vi "Controller & output.vi"() -> ()   [LabVIEW 2016]
doc: "Manually blink and LED attached to a digital output channel of a LINX device by clicking and LED control in LabVIEW."
uses:
  <vilib>/MakerHub/Xbox-One-Controller/Private/Type Defs/Indicators/Controller.ctl
  <vilib>/MakerHub/Xbox-One-Controller/Private/Type Defs/Indicators/A.ctl
  <vilib>/MakerHub/Xbox-One-Controller/Private/Type Defs/Indicators/B.ctl
  <vilib>/MakerHub/Xbox-One-Controller/Private/Type Defs/Indicators/X.ctl
  <vilib>/MakerHub/Xbox-One-Controller/Private/Type Defs/Indicators/Y.ctl
  <vilib>/MakerHub/Xbox-One-Controller/Private/Type Defs/Indicators/Left Bumper.ctl
  <vilib>/MakerHub/Xbox-One-Controller/Private/Type Defs/Indicators/Right Bumper.ctl
  <vilib>/MakerHub/Xbox-One-Controller/Private/Type Defs/Indicators/View.ctl
  <vilib>/MakerHub/Xbox-One-Controller/Private/Type Defs/Indicators/Menu.ctl
  <vilib>/MakerHub/Xbox-One-Controller/Private/Type Defs/Indicators/Thumbstick_Analog.ctl
  <vilib>/MakerHub/Xbox-One-Controller/Private/Type Defs/Indicators/Slider.ctl
  <vilib>/MakerHub/Xbox-One-Controller/Private/Type Defs/Indicators/DPad.ctl
  <vilib>/MakerHub/LINX/Public/Peripherals/Digital/Digital Write 1 Chan.vi
  <vilib>/MakerHub/LINX/Public/Peripherals/Digital/Digital Write N Chans.vi
  <vilib>/MakerHub/LINX/Private/Local IO/LinxDigitalWrite.vi
  <vilib>/MakerHub/LINX/Public/Utilities/Check Channel.vi
  <vilib>/MakerHub/LINX/Public/Utilities/Open Serial.vi
  <vilib>/MakerHub/Xbox-One-Controller/Public/Open First Controller.vi
  <vilib>/MakerHub/LINX/Private/Utilties/Generate Error.vi
  <vilib>/MakerHub/LINX/LMH-LINX.lvlib
  <vilib>/MakerHub/Xbox-One-Controller/LMH-Xbox-One-Controller.lvlib
panel:
  in  "Brake":bool
  in  "DO Channel 2":u8
  in  "y":i32
  out "element":i32
  out "Y Value":i32[](array[numeric])
  out "X value":i32[](array[numeric])
  out "Left Stick":T1
  in  "Frequency (Hz)":u32
  in  "Duration (ms)":u32
  in  "PWM Channel":u8=13
  in  "Stop Button 2":bool
  out "Controller":T2={"A Button"=FALSE, "B Button"=FALSE, "X Button"=FALSE, "Y Button"=FALSE, "Left Bumper"=FALSE, "Right Bumper"=FALSE, "View Button"=FALSE, "Menu Button"=FALSE, "Left Stick"={[], []}, "Right Stick"={[], []}, "Trigger"=0, "D-Pad"=5} {"Trigger" scale=32767.0..-32768.0}
  out "Loop Rate (Hz)":u32
  in  "LED Value":bool
  in  "Digital Output Channel":u8=13
  in  "Serial Port":refnum<visa-resource-name>
  in  "Stop Button":bool
  # "Circuit Schematic"
  # "LINX Device Settings"
  # "Direction"
  # "Manual Blink Example\n\nThis example demonstrates how to blink an LED on a LINX device by clicking on an LED control in LabVIEW.\n\nInstructions\n1. Select the Serial Port associated with the LINX Device.\n2. Select the Digital Output Channel connected to the LED.\n3. Click the Run Arrow."
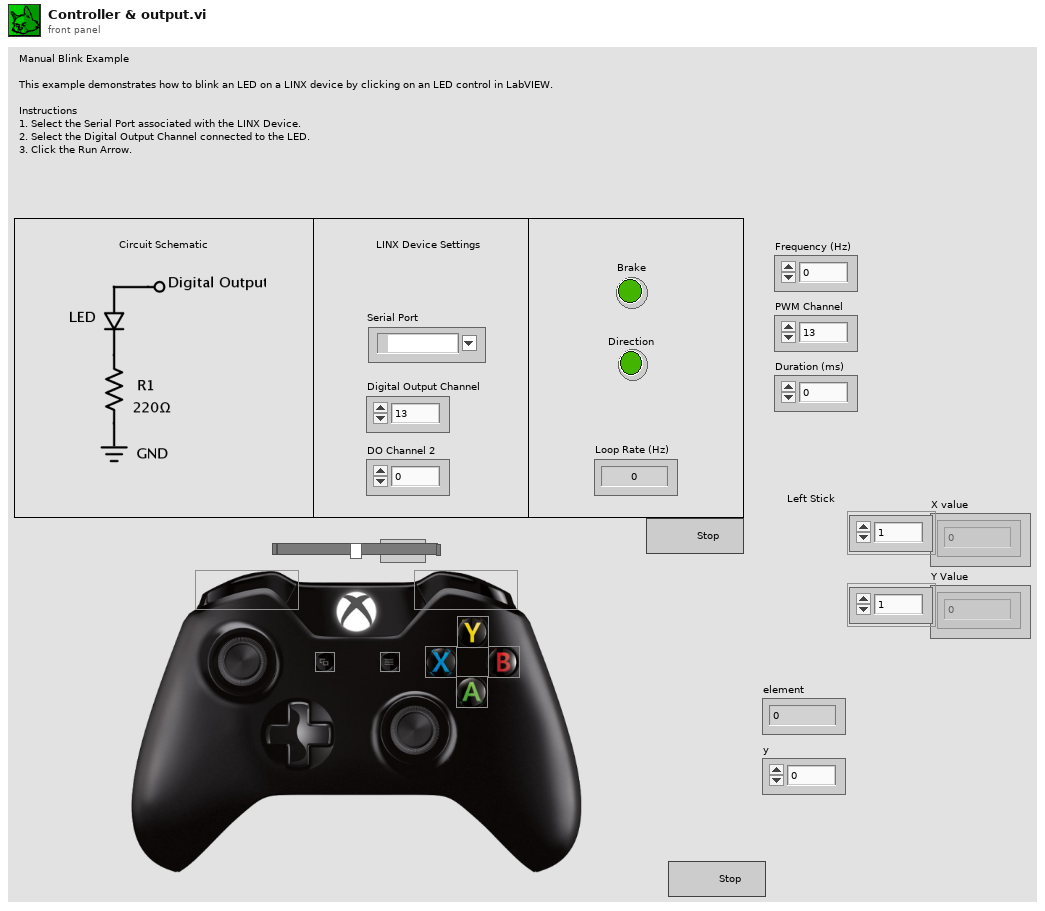
[diagram p1: front panel]
types:
  T1 = typedef "LMH-Xbox-One-Controller.lvlib/Thumbstick_Analog.ctl" = cluster{i32[], i32[]}
  T2 = typedef "LMH-Xbox-One-Controller.lvlib/Controller.ctl" = cluster{"A Button":T3, "B Button":T4, "X Button":T5, "Y Button":T6, "Left Bumper":T7, "Right Bumper":T8, "View Button":T9, "Menu Button":T10, "Left Stick":T1, "Right Stick":T1, "Trigger":T11, "D-Pad":T12}
  T3 = typedef "LMH-Xbox-One-Controller.lvlib/A.ctl" = bool
  T4 = typedef "LMH-Xbox-One-Controller.lvlib/B.ctl" = bool
  T5 = typedef "LMH-Xbox-One-Controller.lvlib/X.ctl" = bool
  T6 = typedef "LMH-Xbox-One-Controller.lvlib/Y.ctl" = bool
  T7 = typedef "LMH-Xbox-One-Controller.lvlib/Left Bumper.ctl" = bool
  T8 = typedef "LMH-Xbox-One-Controller.lvlib/Right Bumper.ctl" = bool
  T9 = typedef "LMH-Xbox-One-Controller.lvlib/View.ctl" = bool
  T10 = typedef "LMH-Xbox-One-Controller.lvlib/Menu.ctl" = bool
  T11 = typedef "LMH-Xbox-One-Controller.lvlib/Slider.ctl" = i32
  T12 = typedef "LMH-Xbox-One-Controller.lvlib/DPad.ctl" = u16
  T13 = typedef "LMH-LINX.lvlib/LINX Ref.ctl" = cluster{"IO":T14, "Interface":T15, "LINX Device Config":T16}
  T14 = typedef "LMH-LINX.lvlib/Platform.ctl" = enum16{"Remote", "Local"}
  T15 = typedef "LMH-LINX.lvlib/Interface.ctl" = enum16{"Serial", "TCP"}
  T16 = typedef "LMH-LINX.lvlib/Device.lvlib/LINX Device Config.ctl" = cluster{"Interface":T15, "COM Port":refnum<visa-resource-name>, "TCP Configuration":T17, "Device Family":u8, "Device ID":u8, "Device Name":string, "TCP Ref":refnum<k5>, "Channels":T18}
  T17 = typedef "LMH-LINX.lvlib/Device.lvlib/TCP Config.ctl" = cluster{"IP Address":string, "Port":u16}
  T18 = typedef "LMH-LINX.lvlib/Channels.ctl" = cluster{"DI":u8[], "DO":u8[], "AI":u8[], "AO":u8[], "PWM":u8[], "QE":u8[], "UART":u8[], "I2C 2":u8[], "SPI":u8[], "CAN":u8[], "Servo":u8[], "AI Ref (V)":dbl, "AI Resolution (Bits)":u8, "AO Ref (V)":dbl, "AO Resolution (Bits)":u8}
  T19 = typedef "LMH-Xbox-One-Controller.lvlib/Xbox One Controller Ref.ctl" = cluster{"Controller Ref":refnum<k1>, "Event Refnum":refnum<event-registration>, "Worker Ref":refnum<vi>}
  T20 = typedef "LMH-Xbox-One-Controller.lvlib/All Axis Data.ctl" = cluster{"Left Stick":cluster{"X Axis":i32, "Y Axis":i32}, "Right Stick":cluster{"X Axis":i32, "Y Axis":i32}, "Triggers":i32, "D-Pad":T21}
  T21 = typedef "LMH-Xbox-One-Controller.lvlib/DPad Enum.ctl" = enum16{"Idle", "Up", "Up / Right", "Right", "Down / Right", "Down", "Down / Left", "Left", "Up / Left"}
  T22 = typedef "LMH-Xbox-One-Controller.lvlib/All Buttons Visual.ctl" = cluster{"A":T3, "B":T4, "X":T5, "Y":T6, "Left Bumper":T7, "Right Bumper":T8, "View Button":T9, "Menu Button":T10, "Left Stick":T23, "Right Stick":T23}
  T23 = typedef "LMH-Xbox-One-Controller.lvlib/Thumbstick.ctl" = bool
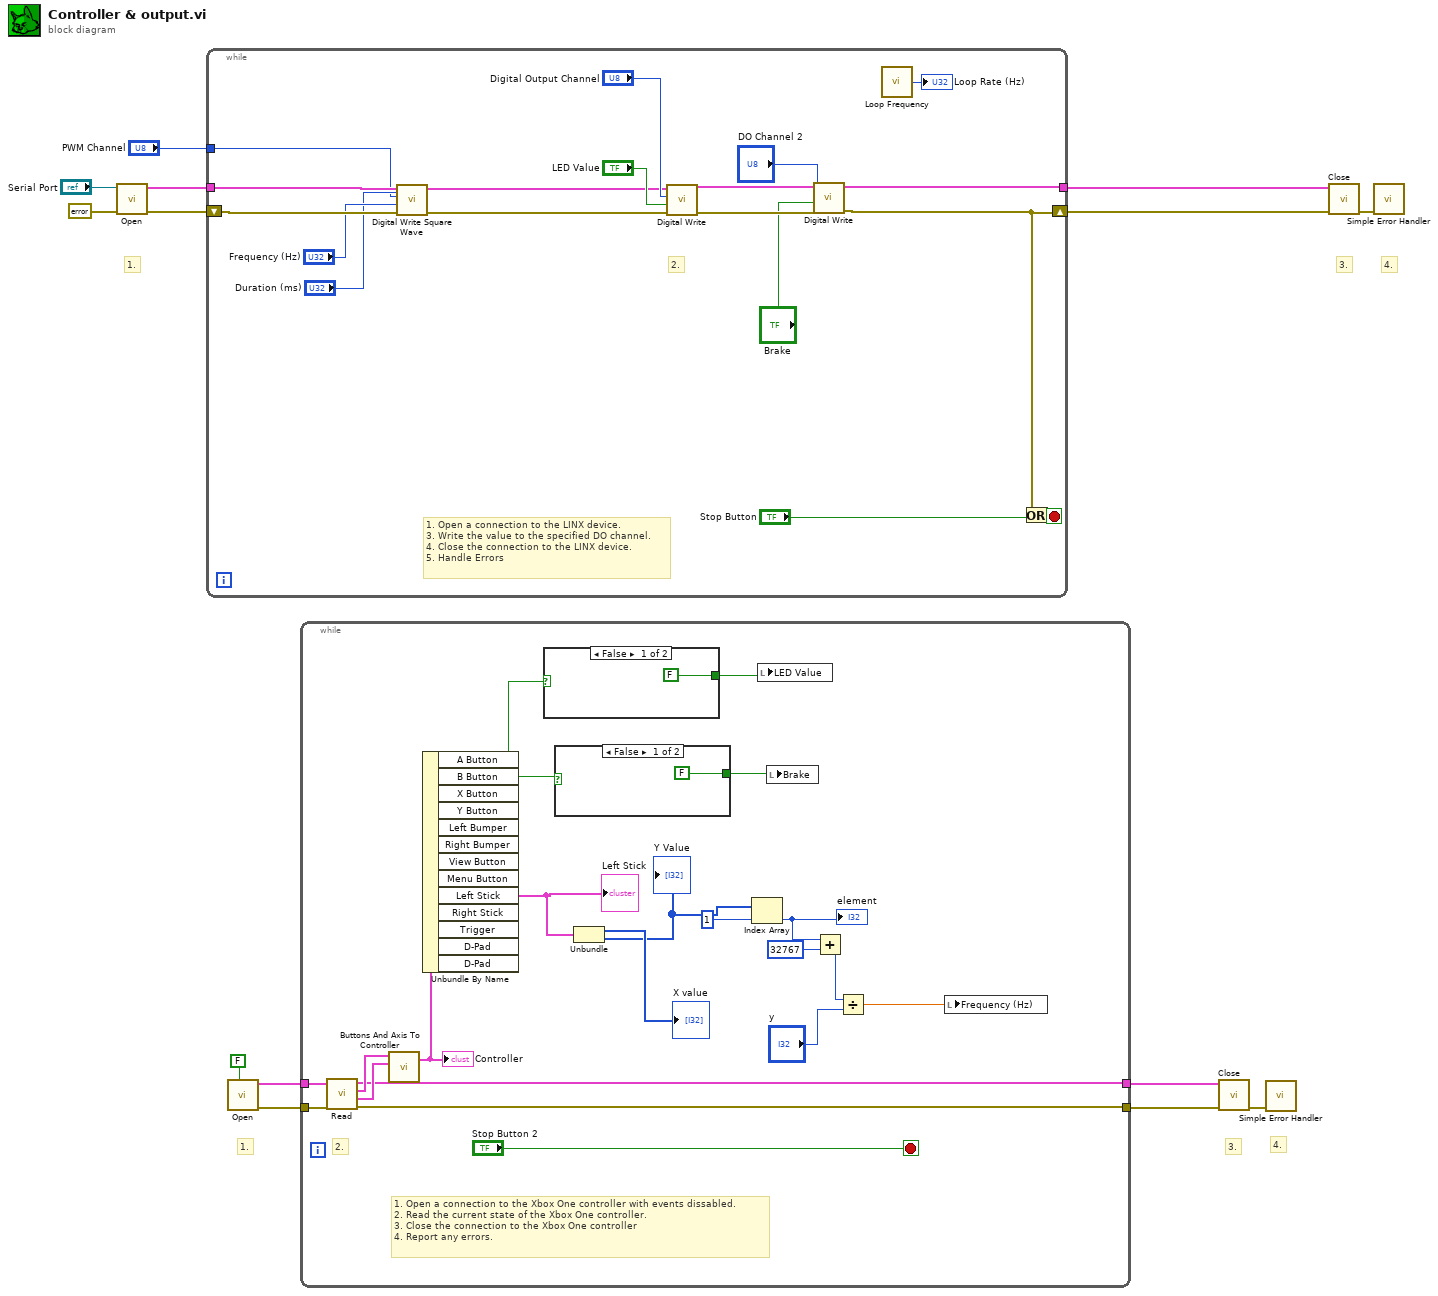
[diagram p0: block diagram]
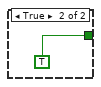
[diagram p2: hidden frame]
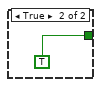
[diagram p3: hidden frame]
diagram:
  # "4."
  # "3."
  # "1."
  # "4."
  # "3."
  # "1."
  n1 = call-poly <vilib>:"Open.vi"("Error In"=errorcluster {"status"=FALSE, "code"=0, "source"=""}, "Serial Port"="Serial Port") -> ("Error Out"=w13:errorcluster, "LINX Resource"=w14:T13)  [unwired: 7 in, 1 out]
  n2 = while {
    tunnel: w14 -> [w24]
    tunnel: [w20] -> w12
    shift-right: [w17] -> w11
    shift-left: w13 -> [w25]
    tunnel: "PWM Channel" -> [w21]
    stop <- w32 stop-if-true
    # "1. Open a connection to the LINX device.\n3. Write the value to the specified DO channel.\n4. Close the connection to the LINX device.\n5. Handle Errors"
    # "2."
    n3 = call <vilib>:"Digital Write Square Wave.vi"("Duration (ms)"="Duration (ms)", "Error In"=w25, "Frequency (Hz)"="Frequency (Hz)", "Channel"=w21, "LINX Resource"=w24) -> ("Error Out"=w26:errorcluster, "LINX Resource"=w27:T13)  [unwired: 5 in]
    n4 = call-poly <vilib>:"Digital Write.vi"("Error In"=w26, "Output Value"="LED Value", "DO Channel"="Digital Output Channel", "LINX Resource"=w27) -> ("Error Out"=w18:errorcluster, "LINX Resource"=w19:T13)  [unwired: 6 in]
    n5 = call-poly <vilib>:"Digital Write.vi"("Error In"=w18, "Output Value"="Brake", "DO Channel"="DO Channel 2", "LINX Resource"=w19) -> ("Error Out"=w17:errorcluster, "LINX Resource"=w20:T13)  [unwired: 6 in]
    n6 = call <vilib>:"Loop Frequency.vi"() -> ("Loop Rate (Hz)"=→"Loop Rate (Hz)":u32)
    n7 = Or(x=w17, y="Stop Button") -> (x .or. y?=w32:bool)
  }
  n8 = call-poly <vilib>:"Open.vi"("Enable Events (T)"=FALSE) -> ("Error Out"=w5:errorcluster, "Xbox One Controller"=w6:T19)  [unwired: 8 in, 1 out]
  n9 = while {
    tunnel: w5 -> [w52]
    tunnel: w6 -> [w47]
    tunnel: [w49] -> w2
    tunnel: [w48] -> w3
    stop <- "Stop Button 2" stop-if-true
    # "1. Open a connection to the Xbox One controller with events dissabled.\n2. Read the current state of the Xbox One controller.\n3. Close the connection to the Xbox One controller\n4. Report any errors."
    # "2."
    n10 = call <vilib>:"Read.vi"("Error In"=w52, "Xbox One Controller Ref"=w47) -> ("Error Out"=w48:errorcluster, "All Axis"=w50:T20, "Buttons"=w51:T22, "Xbox One Controller Ref"=w49:T19)  [unwired: 6 in]
    n11 = call <vilib>:"Buttons And Axis To Controller.vi"("All Axis"=w50, "Buttons"=w51) -> ("Controller"=w46:T2)  [unwired: 5 in]
    "Controller" <- w46
    n12 = Unbundle By Name(w46) -> ("A Button"=w45:T3, "B Button"=w33:T4, "Left Stick"=w43:T1)  [unwired: 10 out]
    "Left Stick" <- w43
    n13 = case shown="False" w45 {
      tunnel: [FALSE ("LED Value") TRUE ("LED Value")] -> w44
      frame False {
      }
      frame True {
      }
    }
    n14 = case shown="False" w33 {
      tunnel: [FALSE ("LED Value") TRUE ("LED Value")] -> w34
      frame False {
      }
      frame True {
      }
    }
    n15 = Unbundle(w43) -> (→"X value":i32[], w41:i32[])
    "Y Value" <- w41
    n16 = Index Array(array=w41, index=1) -> (element=w37:i32)
    "element" <- w37
    n17 = local write "LED Value"(w44) -> ()
    n18 = local write "Brake"(w34) -> ()
    n19 = Add(x=w37, y=32767) -> (x+y=w36:i32)
    n20 = Divide(x=w36, y="y") -> (x/y=w38:ext)
    n21 = local write "Frequency (Hz)"(w38) -> ()
  }
  n22 = call <vilib>:"Close.vi"("Error In"=w3, "Xbox One Controller Ref"=w2) -> ("Error Out"=w4:errorcluster)  [unwired: 9 in]
  n23 = call <vilib>:"Simple Error Handler.vi"("error in (no error)"=w4) -> ()  [unwired: 4 in, 5 out]
  n24 = call <vilib>:"Close.vi"("Error In"=w11, "LINX Resource"=w12) -> ("Error Out"=w9:errorcluster)  [unwired: 9 in]
  n25 = call <vilib>:"Simple Error Handler.vi"("error in (no error)"=w9) -> ()  [unwired: 4 in, 5 out]
